vi "Teleop.vi"(10 "Match Info":T2={"Autonomous Elapsed Seconds"=0.0, "TeleOp Elapsed Seconds"=0.0, "Disabled Elapsed Seconds"=0.0, "Visited Autonomous"=FALSE, "Visited TeleOp"=FALSE, "Visited Disabled"=FALSE, "Autonomous Settings"={"Autonomous Style"=enum."Independent", "VI Refnum"=refnum}}, 11 "Call Context":T3) -> ()   [LabVIEW 2012]
doc: "This VI is called for each TeleOp packet received from the DS where the robot is not disabled. It is often used to read from the joysticks and update I/O or to update setpoints for timed control loops. It should complete and return within 20 milliseconds or it may miss DS packets."
uses:
  <vilib>/Rock Robotics/WPI/DriverStation/WPI_DriverStationDerivedRobotMode.ctl
  <vilib>/Rock Robotics/WPI/DriverStation/WPI_DriverStationMatch Info.ctl
  Robot Global Data.vi
  <vilib>/Rock Robotics/WPI/Joystick/WPI_JoystickGetSetRefNum.vi
panel:
  out "PWM 6 Out":dbl
  out "PWM 5 Out":dbl
  in  "PWM 6":dbl(slide) scale=-1.0..1.0
  in  "PWM 5 (Default)":dbl(slide) scale=-1.0..1.0
  in  "Control Both":bool=TRUE
  in  "Servo Positions":T1={"Shifting"={"Right Servo High"=145.0, "Right Servo Low"=110.0, "Left Servo High"=70.0, "Left Servo Low"=110.0}, "Breaking"={"Coast Position"=0.0, "Break Position"=0.0}}
  # "0.85 - 145"
  # "0.65 - 110"
  # "0.45 - 76"
  # "0.7 - 119"
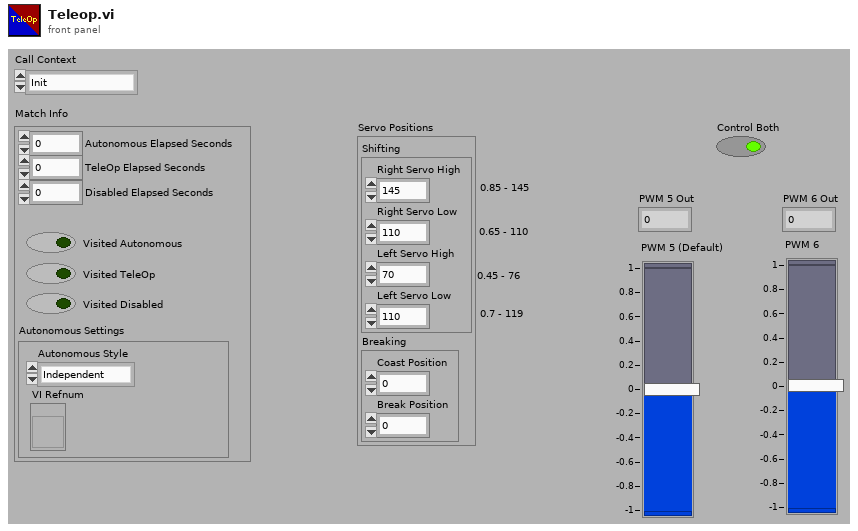
[diagram p1: front panel]
types:
  T1 = cluster{"Shifting":cluster{"Right Servo High":dbl, "Right Servo Low":dbl, "Left Servo High":dbl, "Left Servo Low":dbl}, "Breaking":cluster{"Coast Position":dbl, "Break Position":dbl}}
  T2 = typedef "WPI_DriverStationMatch Info.ctl" = cluster{"Autonomous Elapsed Seconds":dbl, "TeleOp Elapsed Seconds":dbl, "Disabled Elapsed Seconds":dbl, "Visited Autonomous":bool, "Visited TeleOp":bool, "Visited Disabled":bool, "Autonomous Settings":cluster{"Autonomous Style":enum16{"Iterative", "Independent"}, "VI Refnum":refnum<vi>}}
  T3 = typedef "WPI_DriverStationDerivedRobotMode.ctl" = enum16{"Init", "Execute", "Stop"}
  T4 = cluster{"Driver Station Digital Input (1-8)[0]":bool, "Driver Station Digital Input (1-8)[1]":bool, "Driver Station Digital Input (1-8)[2]":bool, "Driver Station Digital Input (1-8)[3]":bool, "Driver Station Digital Input (1-8)[4]":bool, "Driver Station Digital Input (1-8)[5]":bool, "Driver Station Digital Input (1-8)[6]":bool, "Driver Station Digital Input (1-8)[7]":bool, "Driver Station Digital Input (1-8)[8]":bool}
  T5 = typedef "WPI_JoystickDevRef.ctl" = cluster{"Device":T6}
  T6 = typedef "WPI_JoystickDeviceEnum.ctl" = enum16{"USB 1", "USB 2", "USB 3", "USB 4", "Kinect 1", "Kinect 2"}
  T7 = cluster{"axis 1 (x)":dbl, "axis 2 (y)":dbl, "axis 3 (throttle)":dbl, "axis 4":dbl, "axis 5":dbl, "axis 6":dbl}
  T8 = typedef "WPI_MotorControlDeviceRef.ctl" = cluster{"DeviceStatus":errorcluster, "Type":enum16{"PWM", "CAN"}, "PWM":cluster{"Digital Module":T9, "PWM Channel":T10, "DeadBand":T11}, "CAN":cluster{"Device Number":u8, "Control Mode":T12, "Semaphore":T13, "Max Vout":dbl}, "Invert":bool, "TransformRef":T14, "InvTransformRef":T14}
  T9 = typedef "FPGA_TypedefDigitalModule.ctl" = enum16{"Digital Module 1", "Digital Module 2"}
  T10 = typedef "FPGA_DIOPWMChannel.ctl" = enum8{"PWM 1", "PWM 2", "PWM 3", "PWM 4", "PWM 5", "PWM 6", "PWM 7", "PWM 8", "PWM 9", "PWM 10", "Invalid"}
  T11 = typedef "WPI_PWMDeadband.ctl" = cluster{"Name":string, "maxPositivePwm":i32, "minPositivePwm":i32, "centerPwm":i32, "maxNegativePwm":i32, "minNegativePwm":i32, "angularRange":u16}
  T12 = typedef "WPI_CANJaguar_ControlMode.ctl" = enum8{"Percent VBus", "Current", "Speed", "Position", "Voltage"}
  T13 = typedef "Semaphore RefNum" = refnum<k1>
  T14 = typedef "WPI_PWMTransform_ConPane.ctl" = refnum<vi>
  T15 = typedef "WPI_ServoDeviceRef.ctl" = cluster{"DeviceStatus":errorcluster, "Digital Module":T9, "PWM Channel":T10, "DeadBand":T11}
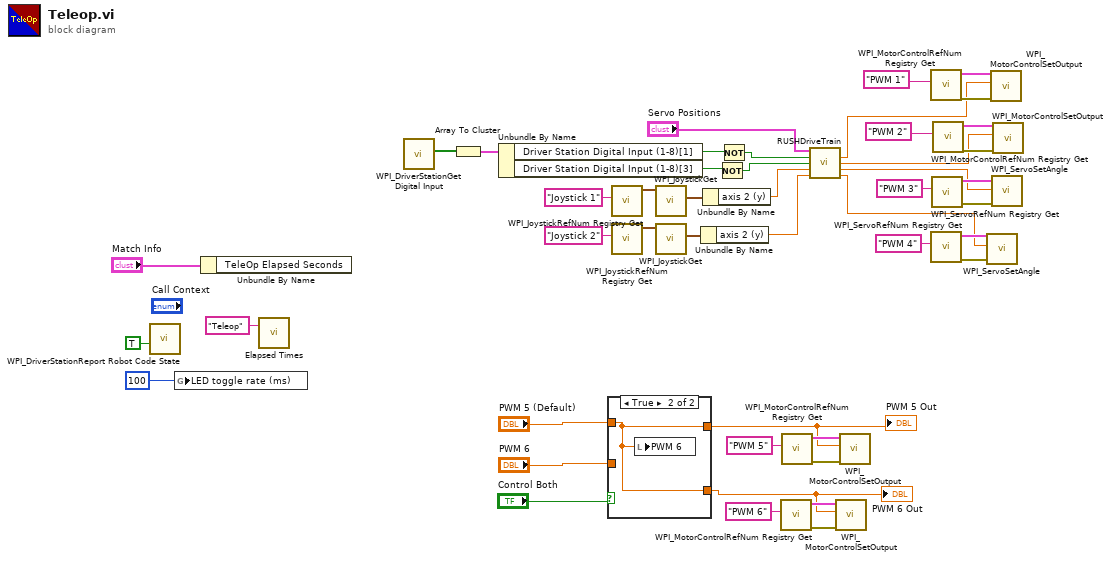
[diagram p0: block diagram]
diagram:
  n1 = call <vilib>:"WPI_DriverStationReport Robot Code State.vi"("TeleOp"=TRUE ("Autonomous")) -> ()  [unwired: 10 in, 1 out]
  n2 = global write "Robot Global Data.vi" "LED toggle rate (ms)"(u32 100 ("LED ms toggle rate")) -> ()
  n3 = Unbundle By Name("Match Info") -> ()  [unwired: 1 out]
  n4 = call "Elapsed Times.vi"("Call Name"="Teleop") -> ()  [unwired: 2 in, 1 out]
  n5 = call <vilib>:"WPI_DriverStationGet Digital Input.vi"() -> ("Driver Station Digital Input (1-8)"=w34:bool[])  [unwired: 11 in]
  n6 = Array To Cluster(array=w34) -> (cluster=w33:T4)
  n7 = Unbundle By Name(w33) -> ("Driver Station Digital Input (1-8)[1]"=w32:bool, "Driver Station Digital Input (1-8)[3]"=w31:bool)
  n8 = case shown="True" "Control Both" {
    tunnel: "PWM 5 (Default)" -> [w47 w49]
    tunnel: "PWM 6" -> [w48 _]
    tunnel: [w48 w49] -> w1
    tunnel: [w47 w49] -> w2
    frame False {
    }
    frame True {
      n9 = local write "PWM 6"(w49) -> ()
    }
  }
  "PWM 6 Out" <- w1
  "PWM 5 Out" <- w2
  n10 = call <vilib>:"WPI_JoystickRefNum Registry Get.vi"("refnum name"="Joystick 1") -> ("JoystickDevRef"=w42:T5)  [unwired: 9 in, 1 out]
  n11 = call <vilib>:"WPI_JoystickRefNum Registry Get.vi"("refnum name"="Joystick 2") -> ("JoystickDevRef"=w39:T5)  [unwired: 9 in, 1 out]
  n12 = call <vilib>:"WPI_JoystickGet.vi"("JoystickDevRef"=w42) -> ("Axes"=w38:T7)  [unwired: 4 in, 2 out]
  n13 = call <vilib>:"WPI_JoystickGet.vi"("JoystickDevRef"=w39) -> ("Axes"=w37:T7)  [unwired: 4 in, 2 out]
  n14 = Unbundle By Name(w37) -> ("axis 2 (y)"=w35:dbl)
  n15 = Unbundle By Name(w38) -> ("axis 2 (y)"=w36:dbl)
  n16 = Not(x=w31) -> (.not. x?=w29:bool)
  n17 = Not(x=w32) -> (.not. x?=w30:bool)
  n18 = call <vilib>:"WPI_MotorControlRefNum Registry Get.vi"("refnum name"="PWM 6") -> ("error out"=w3:errorcluster, "MotorControlDevRef"=w4:T8)  [unwired: 9 in]
  n19 = call <vilib>:"WPI_MotorControlRefNum Registry Get.vi"("refnum name"="PWM 5") -> ("error out"=w5:errorcluster, "MotorControlDevRef"=w6:T8)  [unwired: 9 in]
  n20 = call "RUSHDriveTrain.vi"("Servo Positions"="Servo Positions", "Low Gear + Brake"=w30, "Low Gear"=w29, "LeftJoystick"=w36, "RightJoystick"=w35) -> ("Left Drive"=w20:dbl, "Right Drive"=w19:dbl, "Left Servo"=w15:dbl, "Right Servo"=w12:dbl)  [unwired: 6 in, 1 out]
  n21 = call <vilib>:"WPI_MotorControlSetOutput.vi"("error in (no error)"=w3, "Output"=w1, "MotorControlDevRef"=w4) -> ()  [unwired: 6 in, 3 out]
  n22 = call <vilib>:"WPI_MotorControlSetOutput.vi"("error in (no error)"=w5, "Output"=w2, "MotorControlDevRef"=w6) -> ()  [unwired: 6 in, 3 out]
  n23 = call <vilib>:"WPI_MotorControlRefNum Registry Get.vi"("refnum name"="PWM 1") -> ("error out"=w27:errorcluster, "MotorControlDevRef"=w28:T8)  [unwired: 9 in]
  n24 = call <vilib>:"WPI_ServoRefNum Registry Get.vi"("refnum name"="PWM 4") -> ("error out"=w14:errorcluster, "ServoDeviceRef"=w13:T15)  [unwired: 9 in]
  n25 = call <vilib>:"WPI_ServoRefNum Registry Get.vi"("refnum name"="PWM 3") -> ("error out"=w16:errorcluster, "ServoDeviceRef"=w17:T15)  [unwired: 9 in]
  n26 = call <vilib>:"WPI_MotorControlRefNum Registry Get.vi"("refnum name"="PWM 2") -> ("error out"=w24:errorcluster, "MotorControlDevRef"=w25:T8)  [unwired: 9 in]
  n27 = call <vilib>:"WPI_ServoSetAngle.vi"("error in (no error)"=w14, "Angle"=w12, "ServoDeviceRef"=w13) -> ()  [unwired: 7 in, 2 out]
  n28 = call <vilib>:"WPI_MotorControlSetOutput.vi"("error in (no error)"=w27, "Output"=w20, "MotorControlDevRef"=w28) -> ()  [unwired: 6 in, 3 out]
  n29 = call <vilib>:"WPI_ServoSetAngle.vi"("error in (no error)"=w16, "Angle"=w15, "ServoDeviceRef"=w17) -> ()  [unwired: 7 in, 2 out]
  n30 = call <vilib>:"WPI_MotorControlSetOutput.vi"("error in (no error)"=w24, "Output"=w19, "MotorControlDevRef"=w25) -> ()  [unwired: 6 in, 3 out]
